vi "Returning Values By Reference Pointer To Complex Struct.vi"(11 "triangle":T1) -> (2 "name":string, 3 "triangle out":T1)   [LabVIEW 2018, in "ParsingDataSampleDLL.lvlib"]
doc: "__declspec(dllexport) void ReturningValuesByReference_PointerToComplexStruct (struct complexStructPolygon* triangle);"
uses:
  <vilib>/Utility/importsl/GetValueByPointer/datatype.ctl
  <vilib>/Utility/importsl/GetValueByPointer/GetValueByPointer.xnode
  ParsingDataSampleDLL.lvlib
  ni_reference_vs/Debug/ParsingDataSampleDLL.dll
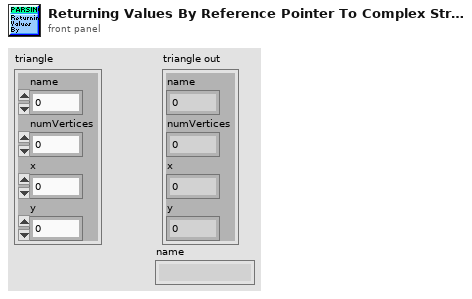
[diagram p1: front panel]
types:
  T1 = cluster{"name":u32, "numVertices":i32, "x":i32, "y":i32}
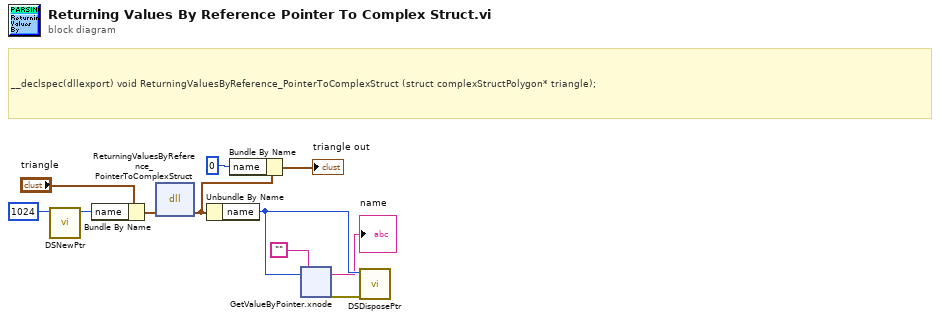
[diagram p0: block diagram]
diagram:
  # "__declspec(dllexport) void ReturningValuesByReference_PointerToComplexStruct (struct complexStructPolygon* triangle);"
  n1 = call <vilib>:"DSNewPtr.vi"("Size"=u64 1024) -> ("Pointer"=w9:u64)  [unwired: 9 in, 1 out]
  n2 = Bundle By Name(cluster="triangle", "name"=w9) -> (w8:T1)
  n3 = dll-call lib="C:/Users/celit/Documents/GitHub/Labview_Python_DLL_Call/ni_reference_vs/Debug/ParsingDataSampleDLL.*" fn="ReturningValuesByReference_PointerToComplexStruct"("triangle"=w8) -> ("triangle"=w3:T1)  [unwired: 4 in, 2 out]
  n4 = Unbundle By Name(w3) -> ("name"=w6:u32)
  n5 = Bundle By Name(cluster=w3, "name"=u32 0) -> (→"triangle out":T1)
  n6 = xnode "GetValueByPointer.xnode"("Pointer"=w6, "InputType"="") -> ("Output"=→"name":string, "ErrorOut"=w7:errorcluster)  [unwired: 2 in]
  n7 = call <vilib>:"DSDisposePtr.vi"("error in (no error)"=w7, "Pointer"=w6) -> ()  [unwired: 9 in, 1 out]
